vi "UART Set Baud Rate.vi"(8 "Error In":errorcluster, 9 "Baud Rate (9600)":u32=9600, 10 "UART Channel":u8, 11 "LINX Device Config":T1) -> (0 "Error Out":errorcluster, 3 "LINX Device Config":T1)   [LabVIEW 2011, in "LVH-LINX.lvlib" / "Device.lvlib"]
doc: "Set the buad rate of the specified UART channel."
uses:
  <vilib>/LabVIEW Hacker/LINX/Private/Device/Device.lvlib
  Type Defs/LINX Device Config.ctl
  Type Defs/Interface.ctl
  Type Defs/TCP Config.ctl
  Type Defs/Device Family.ctl
  Type Defs/Error Type.ctl
  <vilib>/LabVIEW Hacker/LINX/LVH-LINX.lvlib
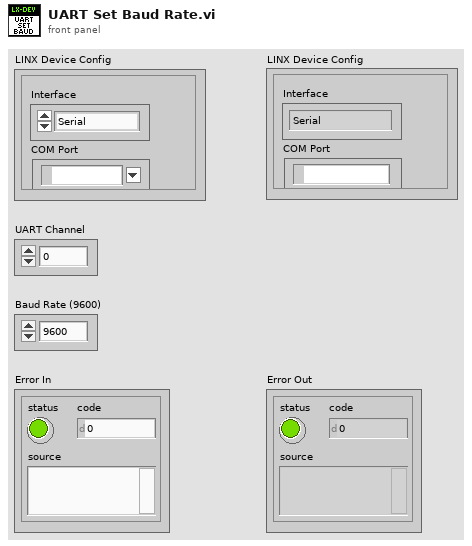
[diagram p1: front panel]
types:
  T1 = typedef "LVH-LINX.lvlib/Device.lvlib/LINX Device Config.ctl" = cluster{"Interface":T2, "COM Port":refnum<visa-resource-name>, "TCP Configuration":T3, "Device ID":u8, "Device Name":string, "Device Family":T4}
  T2 = typedef "LVH-LINX.lvlib/Interface.ctl" = enum16{"Serial", "TCP"}
  T3 = typedef "LVH-LINX.lvlib/Device.lvlib/TCP Config.ctl" = cluster{"IP Address":string, "Port":dbl}
  T4 = typedef "LVH-LINX.lvlib/Device Family.ctl" = enum8{"National Instruments", "Digilent", "Arduino"}
  T5 = typedef "LVH-LINX.lvlib/Error Type.ctl" = enum16{"Unknown", "Timeout", "Corrupt Return Packet", "Unable To Connect", "Command Not Supported", "Channel DNE"}
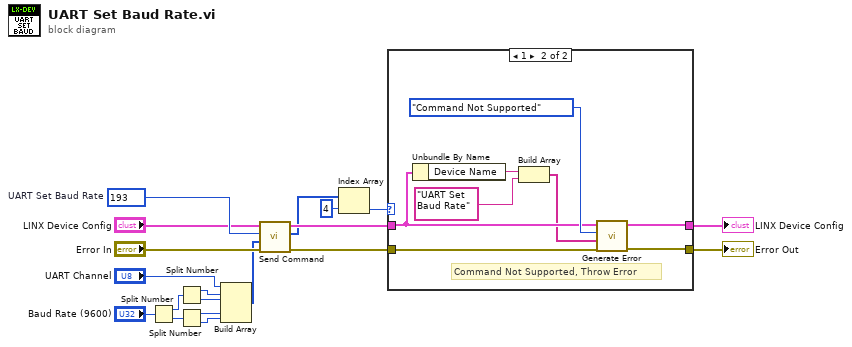
[diagram p0: block diagram]
diagram:
  w18 = u16 193  # UART Set Baud Rate
  n1 = Split Number(x="Baud Rate (9600)") -> (hi(x)=w6:u16, lo(x)=w5:u16)
  n2 = Split Number(x=w6) -> (hi(x)=w4:u8, lo(x)=w3:u8)
  n3 = Split Number(x=w5) -> (hi(x)=w2:u8, lo(x)=w1:u8)
  n4 = Build Array("UART Channel", w4, w3, w2, w1) -> (w8:u8[])
  n5 = call "Send Command.vi"("Error In"="Error In", "ARGS"=w8, "CMD"=w18, "LINX Device Config"="LINX Device Config") -> ("Error Out"=w11:errorcluster, "Response"=w10:u8[], "LINX Device Config"=w13:T1)  [unwired: 5 in]
  n6 = Index Array(array=w10, index=4) -> (element=w15:u8)
  n7 = case shown="1" w15 {
    tunnel: [w21 w27] -> w14
    tunnel: w13 -> [w21 w23]
    tunnel: [w20 w28] -> w12
    tunnel: w11 -> [w20 w29]
    frame 0, Default {
      # "Status OK, Process Data"
    }
    frame 1 {
      # "Command Not Supported, Throw Error"
      n8 = Unbundle By Name(w23) -> ("Device Name"=w25:string)
      n9 = Build Array(w25, "UART Set Baud Rate") -> (w22:string[])
      n10 = call "Generate Error.vi"("Error In"=w29, "Arguments"=w22, "Error Type"=Error_Type."Command Not Supported", "LINX Device Config"=w23) -> ("Error Out"=w28:errorcluster, "LINX Device Config"=w27:T1)  [unwired: 6 in]
    }
  }
  "Error Out" <- w12
  "LINX Device Config" <- w14
